vi "Autonomous Independent.vi"() -> ()   [LabVIEW 2016]
doc: "This VI is called when autonomous begins, and will automatically be terminated when autonomous ends. You can carry out timed or sensor driven robot movement independently without needing to return to the caller."
uses:
  Robot Global Data.vi
  <vilib>/addons/control/pid/pid.llb/PID (DBL).vi
  <vilib>/addons/control/pid/NI_PID_pid.lvlib
  <vilib>/ptbypt/NI_PtbyPt.lvlib
panel:
  out "integral x(t)":dbl format="%0.2f"
  in  "PID gains":T1={"proportional gain (Kc)"=1.0, "integral time (Ti, min)"=0.01, "derivative time (Td, min)"=0.0} {"derivative time (Td, min)" format="%.3f"; "integral time (Ti, min)" format="%.3f"; "proportional gain (Kc)" format="%.3f"}
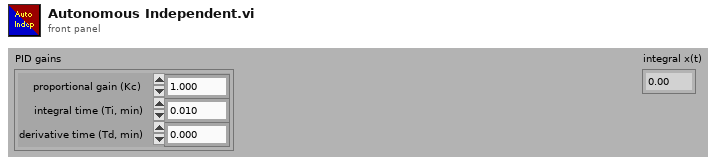
[diagram p1: front panel]
types:
  T1 = cluster{"proportional gain (Kc)":dbl, "integral time (Ti, min)":dbl, "derivative time (Td, min)":dbl}
  T2 = typedef "CTRE_PigeonIMU_DeviceRef.ctl" = cluster{"DeviceStatus":errorcluster, "Device Number":u8, "Type":T3, "Device ID":u32}
  T3 = typedef "CTRE_PigeonIMU_ConnectionType.ctl" = u32
  T4 = typedef "CTRE_PigeonIMU_GlobalStatus.ctl" = cluster{"PigeonState":T5, "FusedHeading":cluster{"Heading":dbl, "Valid?":bool, "Fusing?":bool}, "YPR":cluster{"Yaw":dbl, "Pitch":dbl, "Roll":dbl}, "Compass":cluster{"Heading":dbl, "Magnitude":dbl, "Absolute Heading":dbl}, "Accelerometer":cluster{"Biased":cluster{"X":i16, "Y":i16, "Z":i16, "Norm":i16}, "Angles":cluster{"XZ Tilt":dbl, "YZ Tilt":dbl, "XY Tilt":dbl}}, "Magnetometer":cluster{"Raw":cluster{"X":i16, "Y":i16, "Z":i16}, "Biased":cluster{"X":i16, "Y":i16, "Z":i16}}, "Gyro":cluster{"X":dbl, "Y":dbl, "Z":dbl, "Norm":dbl}, "6D Quaternian":cluster{"W":dbl, "X":dbl, "Y":dbl, "Z":dbl}, "Temp. (C)":dbl, "UpTime":u32, "StartupStatus":cluster{"ResetCount":i32, "ResetFlags":i32, "FirmwareVersion":i32, "HasReset?":bool}, "Calibration":cluster{"CurrentMode":T6, "LastCalError":i32, "CalBooting?":bool}, "CAN Error":errorcluster, "AccumGyro":cluster{"X":dbl, "Y":dbl, "Z":dbl}, "Usage Frame":u32}
  T5 = typedef "CTRE_PigeonIMU_PigeonState.ctl" = enum16{"NoComm", "Initializing", "Ready", "UserCalibration"}
  T6 = typedef "CTRE_PigeonIMU_CalibrationMode.ctl" = u16
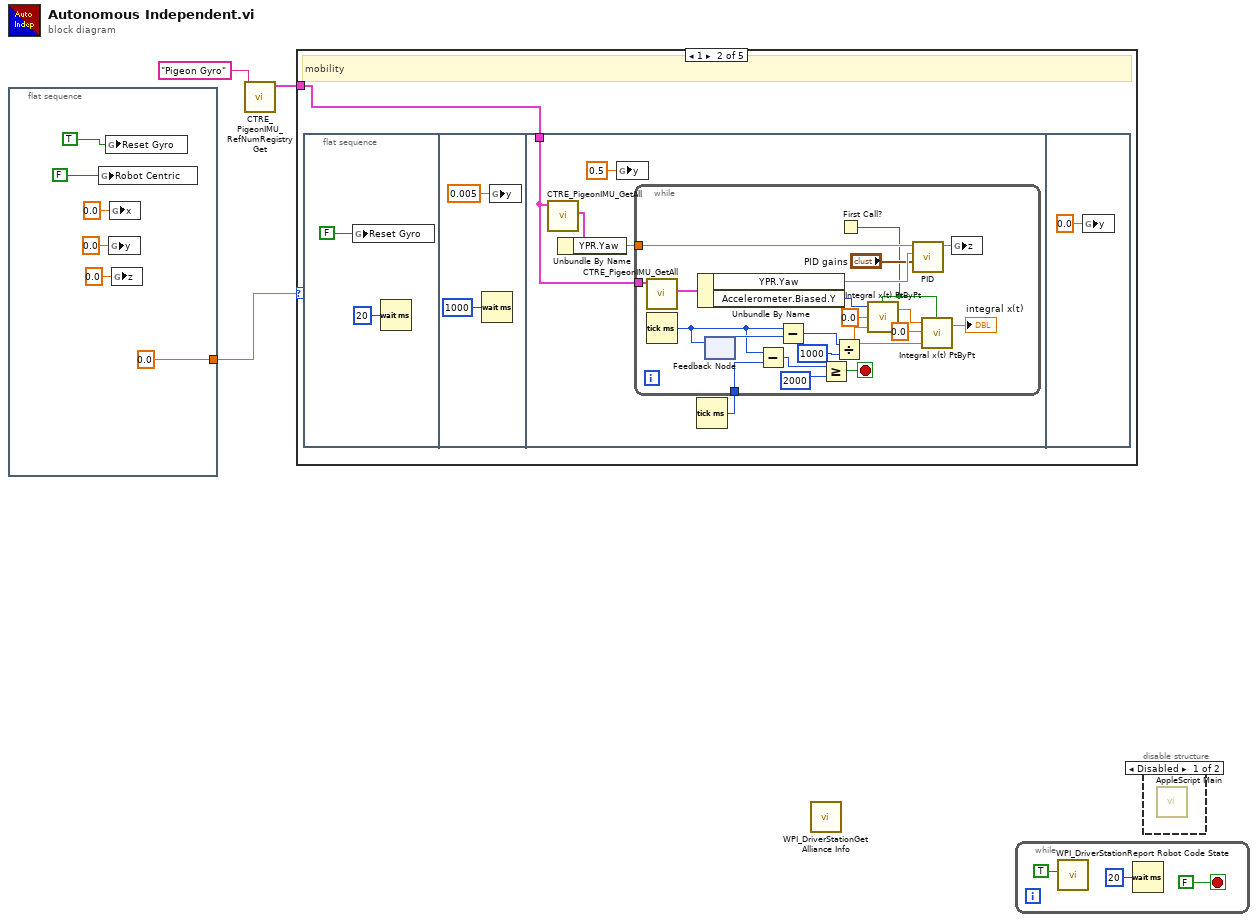
[diagram p0: block diagram]
diagram:
  n1 = flat-sequence {
    tunnel: [0.0 ("Numeric")] -> w2
    frame #0 {
      n2 = global write "Robot Global Data.vi" "Robot Centric"(FALSE) -> ()
      n3 = global write "Robot Global Data.vi" "Reset Gyro"(TRUE) -> ()
      n4 = global write "Robot Global Data.vi" "y"(0.0 ("y")) -> ()
      n5 = global write "Robot Global Data.vi" "x"(0.0 ("x")) -> ()
      n6 = global write "Robot Global Data.vi" "z"(0.0 ("z")) -> ()
    }
  }
  n7 = call <vilib>:"CTRE_PigeonIMU_RefNumRegistryGet.vi"("refnum name"="Pigeon Gyro") -> ("PigeonIMUDevRef"=w1:T2)  [unwired: 9 in, 1 out]
  n8 = case shown="1" w2 {
    tunnel: w1 -> [_ w10 _ _ _]
    frame 0, Default {
      # "Do nothing"
    }
    frame 1 {
      # "mobility"
      n9 = flat-sequence {
        tunnel: w10 -> [w17]
        frame #0 {
          n10 = global write "Robot Global Data.vi" "Reset Gyro"(FALSE) -> ()
          n11 = Wait (ms)(milliseconds to wait=u32 20) -> ()  [unwired: 1 out]
        }
        frame #1 {
          n12 = Wait (ms)(milliseconds to wait=u32 1000) -> ()  [unwired: 1 out]
          n13 = global write "Robot Global Data.vi" "y"(0.005 ("y")) -> ()
        }
        frame #2 {
          n14 = call <vilib>:"CTRE_PigeonIMU_GetAll.vi"("PigeonIMUDevRef"=w17) -> ("Get All"=w18:T4)  [unwired: 8 in, 2 out]
          n15 = Unbundle By Name(w18) -> ("YPR.Yaw"=w16:dbl)
          n16 = global write "Robot Global Data.vi" "y"(0.5 ("y")) -> ()
          n17 = Tick Count (ms)() -> (millisecond timer value=w15:u32)
          n18 = while {
            tunnel: w17 -> [w37]
            tunnel: w16 -> [w35]
            tunnel: w15 -> [w25]
            stop <- w39 stop-if-true
            n19 = call <vilib>:"CTRE_PigeonIMU_GetAll.vi"("PigeonIMUDevRef"=w37) -> ("Get All"=w38:T4)  [unwired: 8 in, 2 out]
            n20 = Tick Count (ms)() -> (millisecond timer value=w29:u32)
            n21 = Unbundle By Name(w38) -> ("YPR.Yaw"=w36:dbl, "Accelerometer.Biased.Y"=w31:i16)
            n22 = feedback-in #1(w29) -> ()
            n23 = feedback #1() -> (w30:u32)  [unwired: 1 in]
            n24 = Subtract(x=w29, y=w25) -> (x-y=w26:u32)
            n25 = Subtract(x=w29, y=w30) -> (x-y=w28:u32)
            n26 = Greater Or Equal?(x=w26, y=u32 2000 ("milliseconds to wait")) -> (x >= y?=w39:bool)
            n27 = Divide(x=w28, y=u32 1000) -> (x/y=w23:dbl)
            n28 = First Call?() -> (First Call?: T/F=w20:bool)
            n29 = call <vilib>:"Integral x(t) PtByPt.vi"("initialize"=w20, "dt"=w23, "initial condition"=0.0, "x"=w31) -> ("integral x(t)"=w32:dbl)  [unwired: 1 out]
            n30 = call-poly <vilib>:"PID.vi"("PID gains"="PID gains", "process variable"=w36, "setpoint"=w35) -> ("output"=w34:dbl)  [unwired: 7 in, 1 out]
            n31 = call <vilib>:"Integral x(t) PtByPt.vi"("initialize"=w20, "dt"=w23, "initial condition"=0.0, "x"=w32) -> ("integral x(t)"=→"integral x(t)":dbl)  [unwired: 1 out]
            n32 = global write "Robot Global Data.vi" "z"(w34) -> ()
          }
        }
        frame #3 {
          n33 = global write "Robot Global Data.vi" "y"(0.0 ("y")) -> ()
        }
      }
    }
    frame 2 {
      # "maybe gear?"
    }
    frame 3 {
      # "maybe left gear?"
    }
    frame 4 {
      # "maybe right gear?"
    }
  }
  n34 = call <vilib>:"WPI_DriverStationGet Alliance Info.vi"() -> ()  [unwired: 12 out]
  n35 = while {
    stop <- FALSE stop-if-true
    n36 = call <vilib>:"WPI_DriverStationReport Robot Code State.vi"("Autonomous"=TRUE) -> ()  [unwired: 10 in, 1 out]
    n37 = Wait (ms)(milliseconds to wait=u32 20) -> ()  [unwired: 1 out]
  }
  n38 = disable-structure shown="Disabled" {
    frame Disabled {
      n39 = call "AppleScript Main.vi"() -> ()  [unwired: 12 in]
    }
    frame Enabled {
    }
  }
